vi "gas flow controller -- Pgg2.vi"(5 "gas flow, %":dbl=11.0, 6 "action":T3=enum."stop UP/DOWN", 7 "heater":dbl=11.0, 8 "gas flow controller ref":refnum<vi>, 10 "seconds":dbl=1.0) -> (0 "gas flow controller out":T1={"DOWN step (%)"=3.0, "below"=TRUE, "above"=FALSE, "check (min)"=11.0, "upper"=12.0, "lower"=3.0, "in range"=FALSE, "ramp step (%)"=0.1, "DOWN time (min)"=60.0, "UP time (min)"=60.0, "UP step (%)"=3.0, "set gas"=FALSE, "to"=90.0, "ramp UP"=FALSE, "ramp DOWN"=FALSE, "idle"=FALSE, "Control Gas"=TRUE, "state"=enum."ramp down", "ramp Up progress"={"(total # of ramp steps)"=30, "ramp time step (sec)"=120, "steps so far"=0, "state"=enum."ramp down"}, "ramp Down progress"={"(total # of ramp steps)"=30, "ramp time step (sec)"=120, "steps so far"=0, "state"=enum."ramp down"}, "last (min)"=90.0, "heater"=90.0, "gas, %"=90.0} {"last (min)" format="%3.3f"})   [LabVIEW 2014]
uses:
  gas flow controller action.ctl
  gas flow controller control.ctl
  gas flow control - progress.ctl
  gas flow controller state.ctl
  stack action -- control.ctl
  itc 503 box - control.ctl
  Q - not nan -- real.vi
  Q - not nan -- integer.vi
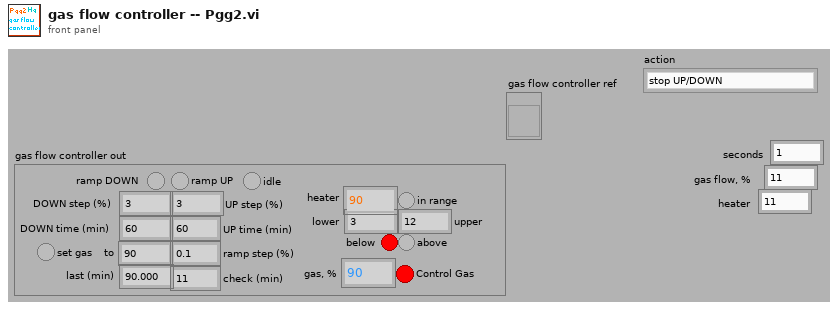
[diagram p1: front panel]
types:
  T1 = typedef "gas flow controller control.ctl" = cluster{"DOWN step (%)":dbl, "below":bool, "above":bool, "check (min)":dbl, "upper":dbl, "lower":dbl, "in range":bool, "ramp step (%)":dbl, "DOWN time (min)":dbl, "UP time (min)":dbl, "UP step (%)":dbl, "set gas":bool, "to":dbl, "ramp UP":bool, "ramp DOWN":bool, "idle":bool, "Control Gas":bool, "state":enum16{"normal", "ramp up", "ramp down"}, "ramp Up progress":T2, "ramp Down progress":T2, "last (min)":dbl, "heater":dbl, "gas, %":dbl}
  T2 = typedef "gas flow control - progress.ctl" = cluster{"(total # of ramp steps)":i32, "ramp time step (sec)":i32, "steps so far":i32, "state":enum16{"normal", "ramp up", "ramp down"}}
  T3 = typedef "gas flow controller action.ctl" = enum16{"check", "force UP", "stop UP/DOWN", "force DOWN", "init", "set gas to", "turn off", "turn on", "idle", "update parameters", "parse", "set gas"}
  T4 = typedef "gas flow controller state.ctl" = enum16{"normal", "ramp up", "ramp down"}
  T5 = typedef "stack action -- control.ctl" = enum16{"push", "pop", "check", "init"}
  T6 = typedef "itc 503 box - control.ctl" = enum16{"heater manual and zero", "heater auto", "upload D", "upload I", "upload P", "shut off", "init", "read sweep table", "disable", "enable", "read state", "set gas to", "stop sweep", "start sweep", "test", "set temperature to", "write sweep table", "-void", "set heater to"}
  T7 = typedef "comparison control.ctl" = enum16{"not a number", "above", "in range", "below"}
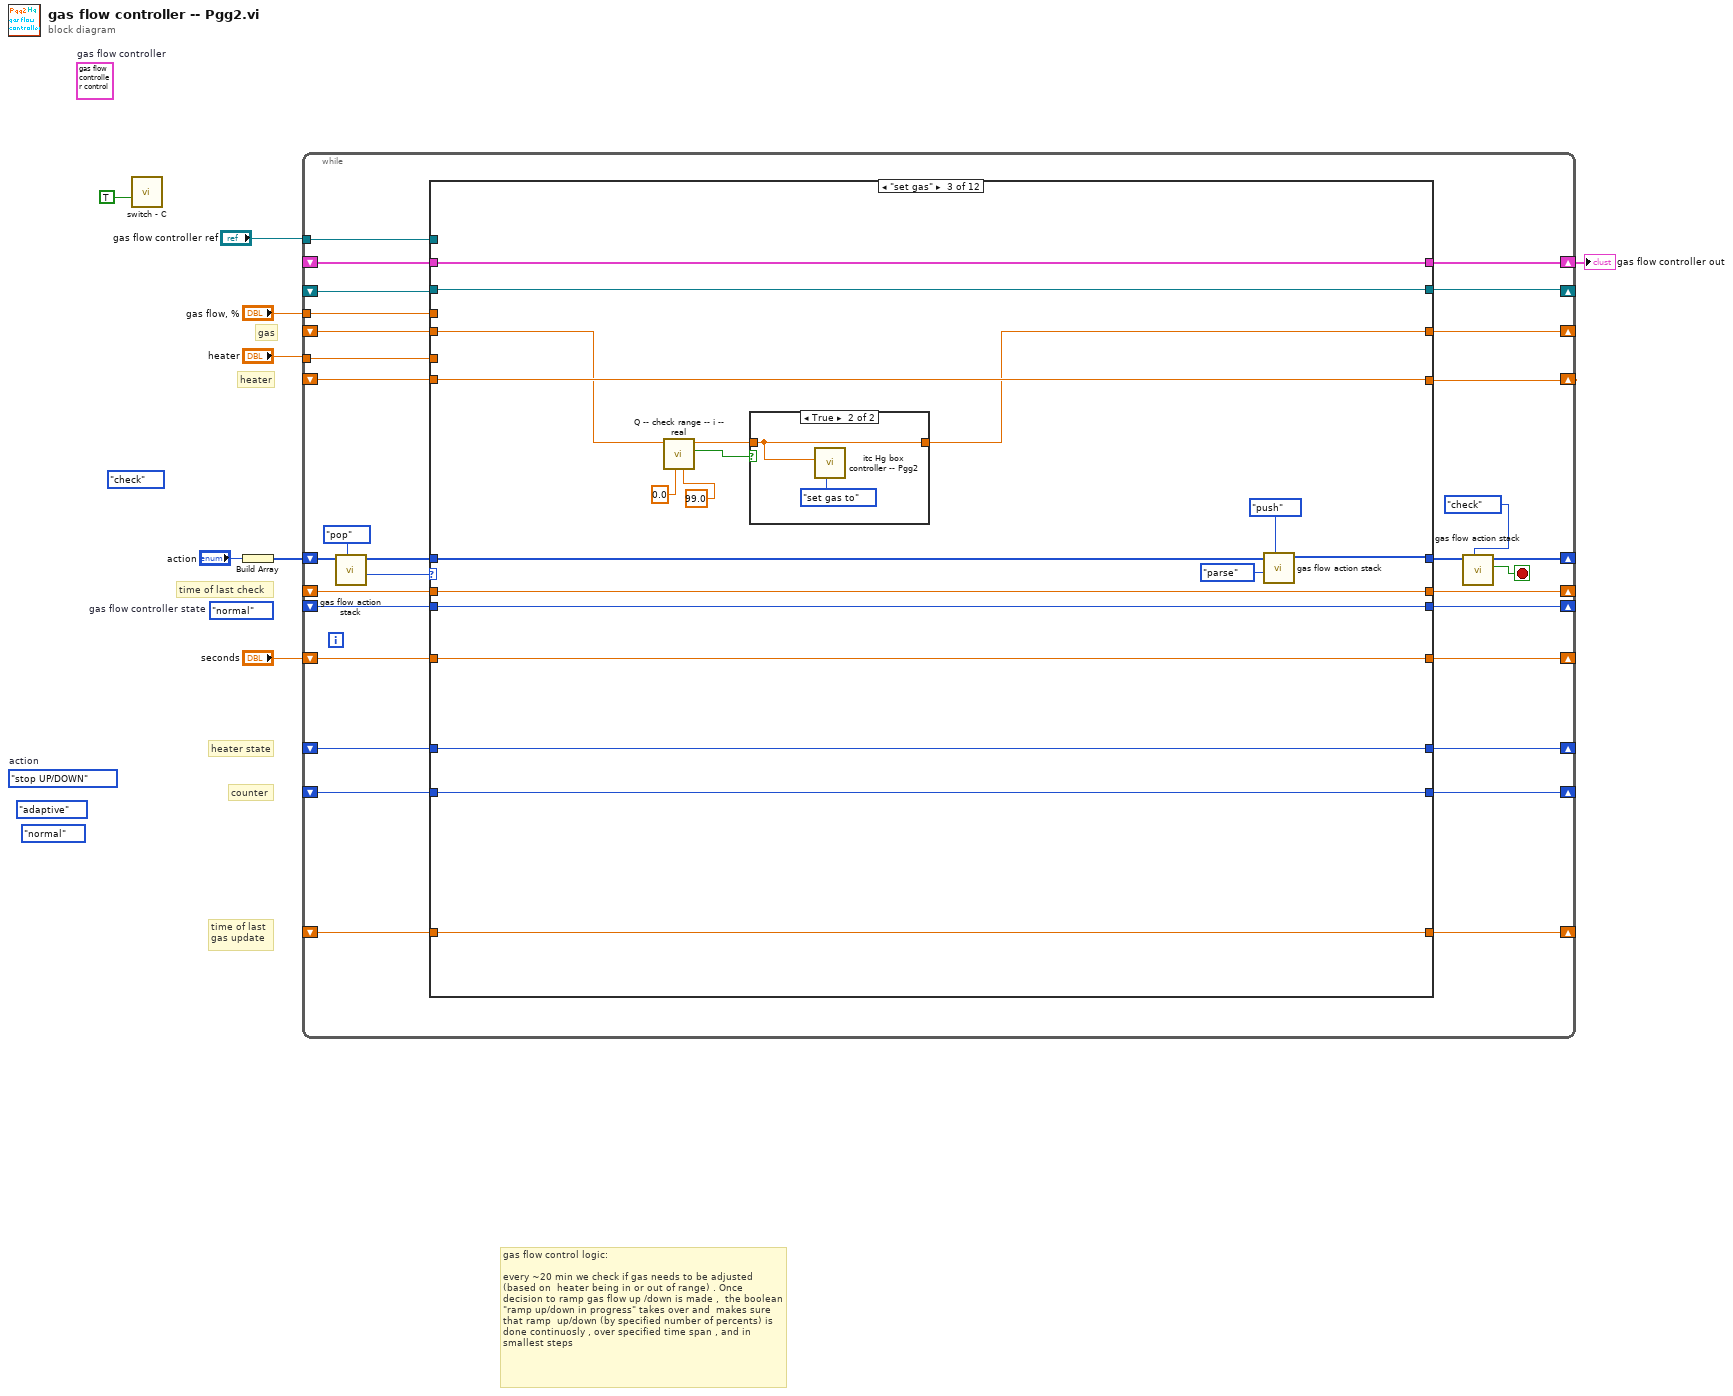
[diagram p0: block diagram]
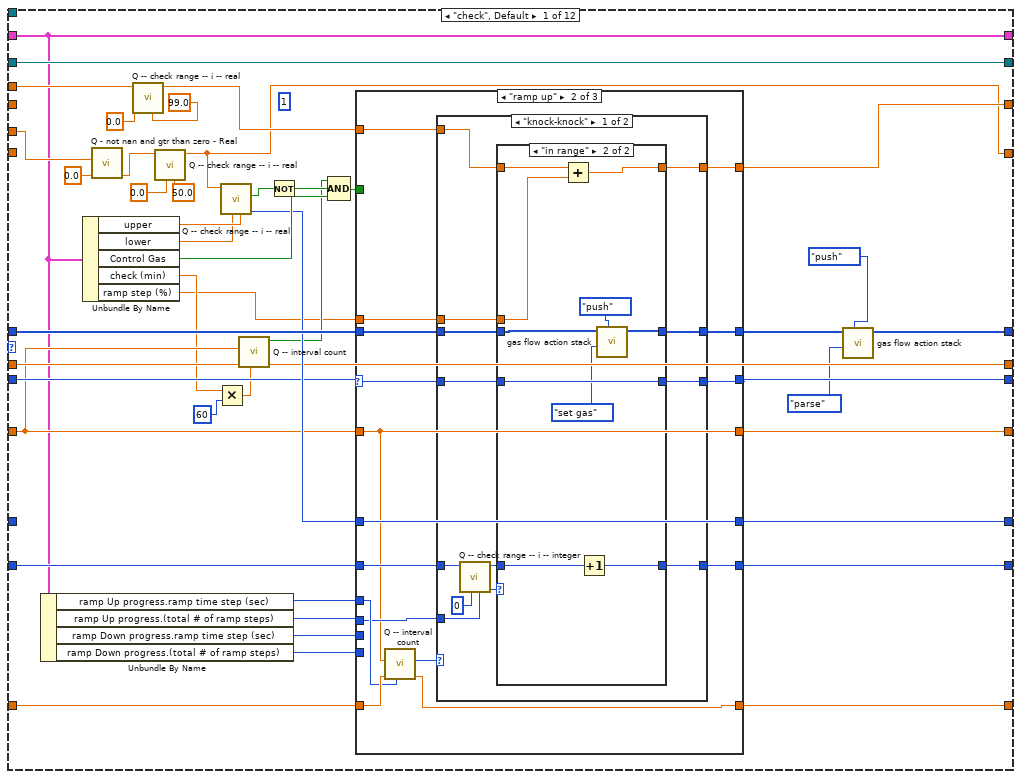
[diagram p2: hidden frame]
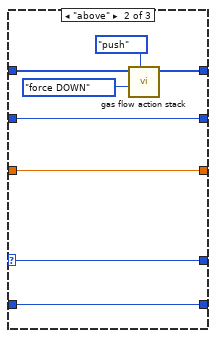
[diagram p5: hidden frame]
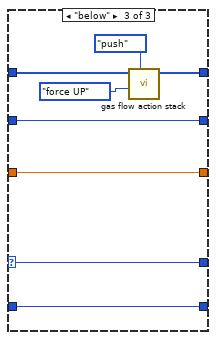
[diagram p6: hidden frame]
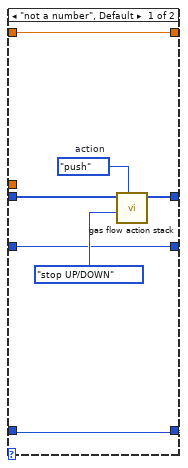
[diagram p7: hidden frame]
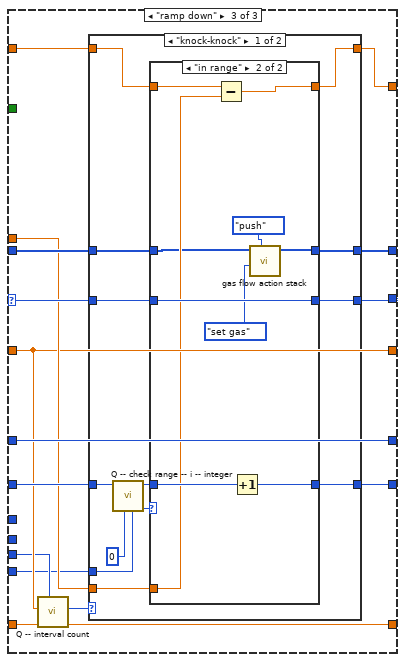
[diagram p9: hidden frame]
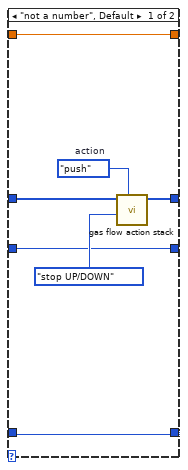
[diagram p10: hidden frame]
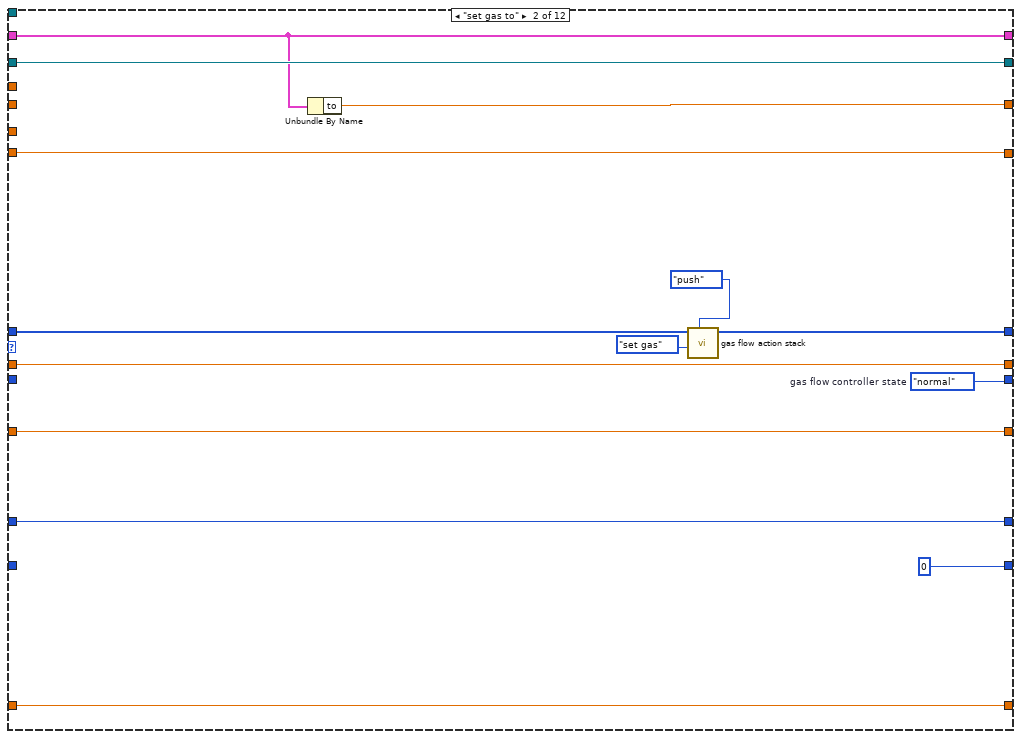
[diagram p12: hidden frame]
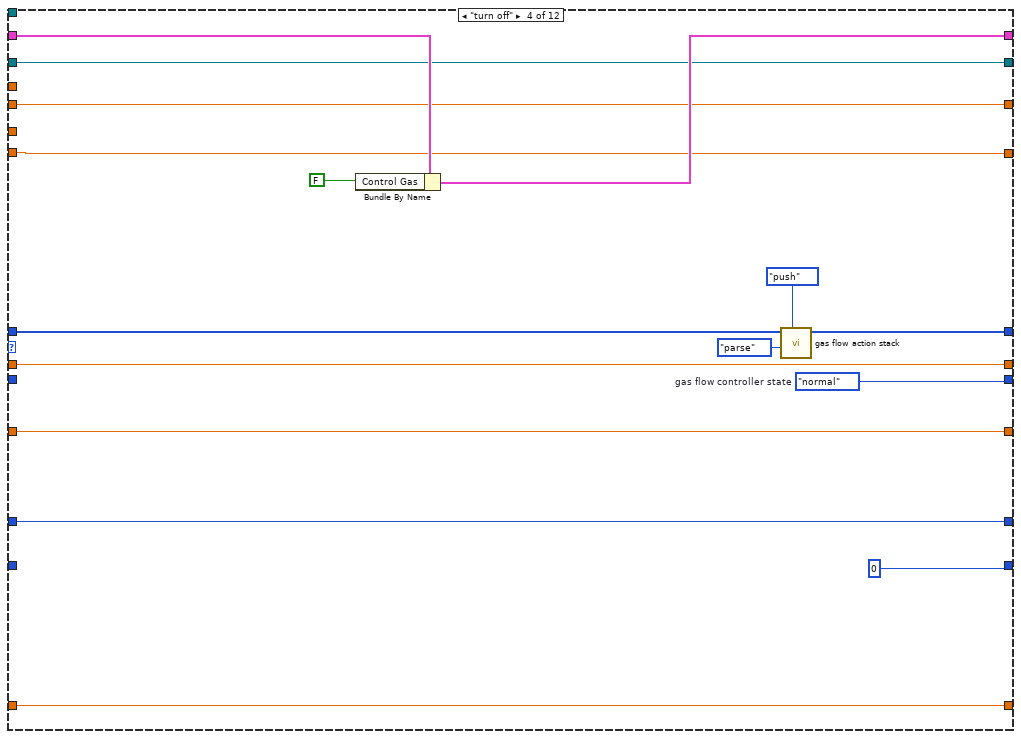
[diagram p14: hidden frame]
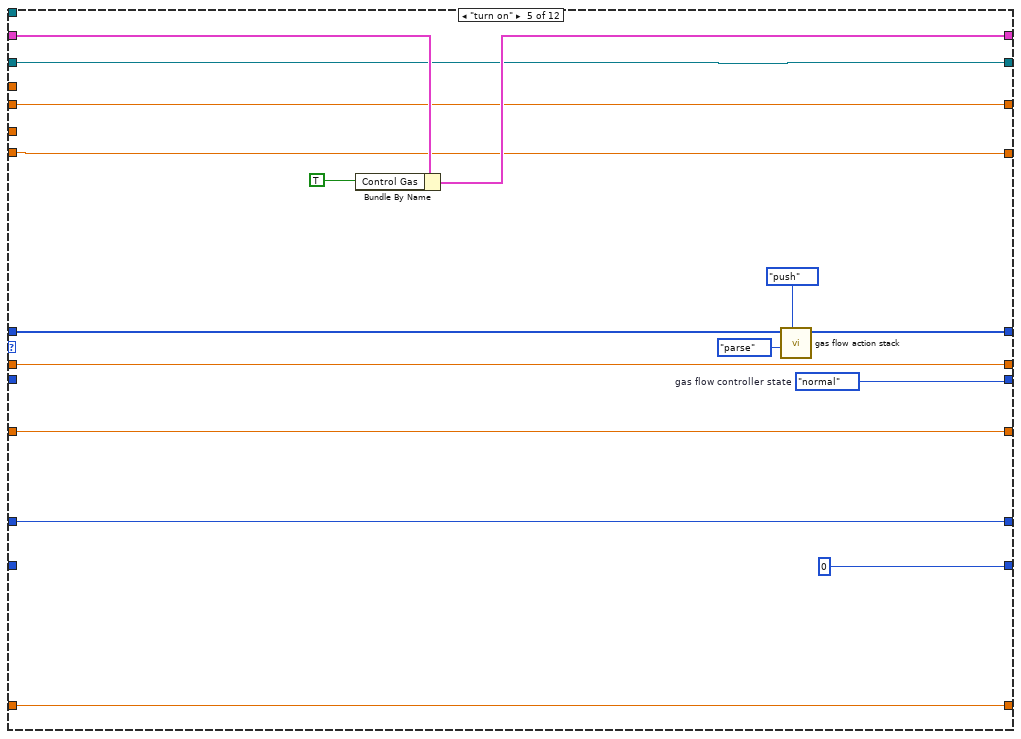
[diagram p15: hidden frame]
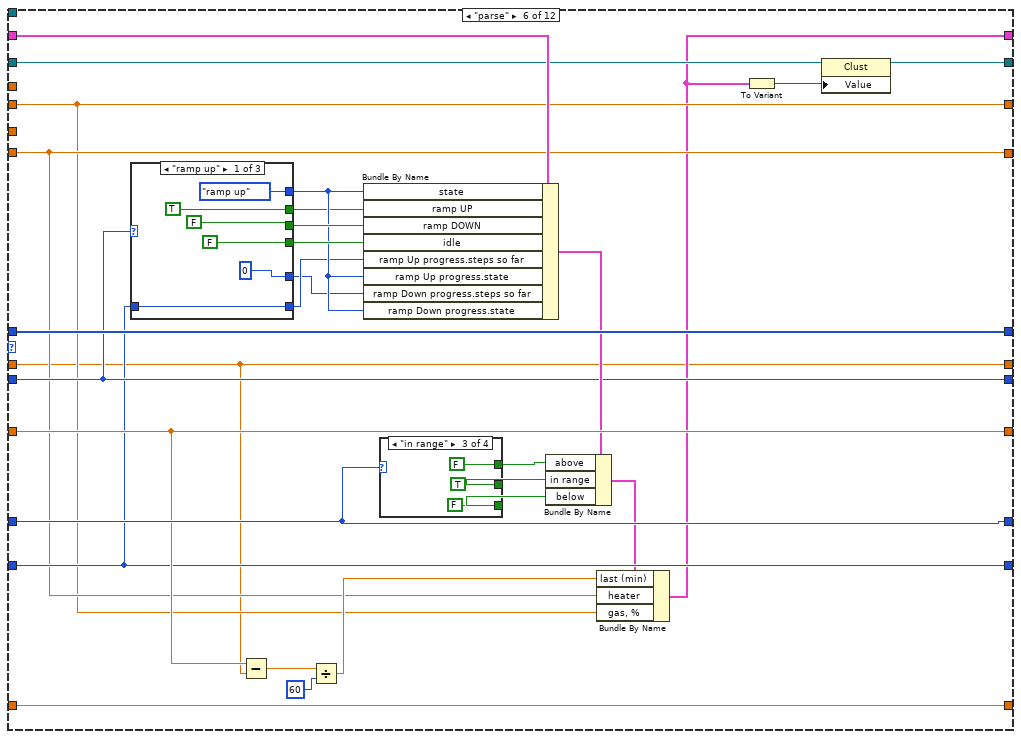
[diagram p16: hidden frame]
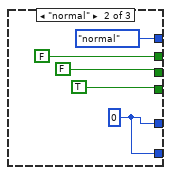
[diagram p17: hidden frame]
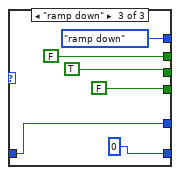
[diagram p18: hidden frame]
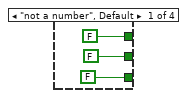
[diagram p19: hidden frame]
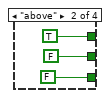
[diagram p20: hidden frame]
diagram:
  (unwired) gas_flow_controller_action."check" ("action")
  (unwired) T1 {"DOWN step (%)"=0.0, "below"=FALSE, "above"=FALSE, "check (min)"=0.0, "upper"=0.0, "lower"=0.0, "in range"=FALSE, "ramp step (%)"=0.0, "DOWN time (min)"=0.0, "UP time (min)"=0.0, "UP step (%)"=0.0, "set gas"=FALSE, "to"=0.0, "ramp UP"=FALSE, "ramp DOWN"=FALSE, "idle"=FALSE, "Control Gas"=FALSE, "state"=enum."normal", "ramp Up progress"={"(total # of ramp steps)"=0, "ramp time step (sec)"=0, "steps so far"=0, "state"=enum."normal"}, "ramp Down progress"={"(total # of ramp steps)"=0, "ramp time step (sec)"=0, "steps so far"=0, "state"=enum."normal"}, "last (min)"=0.0, "heater"=0.0, "gas, %"=0.0}  # gas flow controller
  (unwired) enum16{"normal", "ramp up", "ramp down"}."normal" ("state")
  (unwired) enum16{"first time", "uniform", "adaptive"}."adaptive" ("mode")
  (unwired) gas_flow_controller_state."normal"  # gas flow controller state
  (unwired) gas_flow_controller_action."stop UP/DOWN"  # action
  # "heater"
  # "time of last\ngas update"
  # "counter"
  # "heater state"
  # "gas"
  # "gas flow control logic: \n\nevery ~20 min we check if gas needs to be adjusted  (based on  heater being in or out of range) . Once  decision to ramp gas flow up /down is made ,  the boolean \"ramp up/down in progress\" takes over and  makes sure that ramp  up/down (by specified number of percents) is done continuosly , over specified time span , and in smallest steps"
  # "time of last check"
  n1 = call "switch - C.vi"("switch"=TRUE) -> ()  [unwired: 10 in, 1 out]
  n2 = Build Array("action") -> (w4:T3[])
  n3 = while {
    shift-right: [w39] -> w3
    shift-left: _ -> [w38]
    shift-right: [w20] -> _
    shift-left: _ -> [w17]
    tunnel: "gas flow, %" -> [w21]
    tunnel: "heater" -> [w37]
    shift-right: [w35] -> _
    shift-left: _ -> [w34]
    shift-right: [w33] -> _
    shift-left: _ -> [w32]
    shift-right: [w26] -> _
    shift-left: w4 -> [w31]
    shift-right: [w22] -> _
    shift-left: _ -> [w23]
    shift-right: [w19] -> _
    shift-left: _ -> [w18]
    shift-right: [w15] -> _
    shift-left: "seconds" -> [w36]
    shift-right: [w16] -> _
    shift-left: _ -> [w10]
    shift-right: [w14] -> _
    shift-left: _ -> [w13]
    shift-right: [w12] -> _
    shift-left: _ -> [w11]
    tunnel: "gas flow controller ref" -> [w9]
    stop <- w24 stop-if-true
    n4 = call "gas flow action stack.vi"("action"=stack_action_--_control."pop", "command stack"=w31) -> ("selector out"=w30:T3, "command stack out"=w28:T3[])  [unwired: 7 in, 1 out]
    n5 = case shown="\"set gas\"" w30 {
      tunnel: [w42 w236 w264 w281 w297 w304 w364 w411 w416 w437 w454 w469] -> w39
      tunnel: w38 -> [w42 w236 w264 w284 w300 w322 w369 w411 _ w437 w454 w469]
      tunnel: w37 -> [w47 _ _ _ _ _ _ _ _ _ _ _]
      tunnel: w36 -> [w64 w239 w262 w274 w290 w325 w375 w408 w421 w438 w443 w461]
      tunnel: [w53 w247 w266 w270 w286 w328 w380 w412 w420 w436 w455 w470] -> w35
      tunnel: w34 -> [w53 w247 w266 w270 w286 w306 w368 w412 _ w436 w455 w470]
      tunnel: [w73 w246 w265 w283 w299 w302 w378 w415 w431 w442 w445 w459] -> w33
      tunnel: w32 -> [w75 w246 w265 w283 w299 w302 w378 w415 w431 w442 _ _]
      tunnel: [w57 w243 w257 w279 w295 w329 w377 w403 w424 w435 w448 w463] -> w27
      tunnel: w28 -> [w78 w235 w256 w278 w294 w329 w377 w404 w425 w435 w449 w464]
      tunnel: w23 -> [w76 _ w254 _ _ w315 w376 _ _ w432 _ _]
      tunnel: [w70 w245 w254 w282 w298 w315 w376 w414 w430 w432 w457 w472] -> w22
      tunnel: w21 -> [w69 _ _ _ _ _ _ _ _ _ _ _]
      tunnel: [w49 w244 w248 w276 w292 w307 w370 w410 w428 w441 w453 w468] -> w20
      tunnel: [w48 w240 w263 w275 w291 w308 w371 w409 w427 w440 w452 w467] -> w19
      tunnel: w18 -> [_ w240 w263 w275 w291 w308 w371 w409 w427 w440 w452 w467]
      tunnel: w17 -> [_ _ w250 w276 w292 w307 w370 w410 w428 w441 w453 w468]
      tunnel: [w54 w238 w261 w273 w289 w327 w374 w407 w422 w439 w451 w466] -> w16
      tunnel: [w55 w239 w262 w274 w290 w325 w375 w408 w421 w438 w443 w461] -> w15
      tunnel: [w63 w237 w259 w272 w288 w326 w372 w405 w421 w434 w445 w459] -> w14
      tunnel: w13 -> [w62 w237 w259 w272 w288 w326 w372 w405 _ w434 w444 w458]
      tunnel: [w61 0 w260 0 0 w312 w373 0 0 w433 0 0] -> w12
      tunnel: w11 -> [w60 _ w260 _ _ w312 w373 _ _ w433 _ _]
      tunnel: w10 -> [_ w238 w261 w273 w289 w327 w374 w407 w422 w439 w451 w466]
      tunnel: w9 -> [_ _ _ _ _ _ _ _ w419 _ _ _]
      frame "check", Default {
        (unwired) 1
        n6 = Unbundle By Name(w42) -> ("ramp Up progress.ramp time step (sec)"=w52:i32, "ramp Up progress.(total # of ramp steps)"=w51:i32, "ramp Down progress.ramp time step (sec)"=w44:i32, "ramp Down progress.(total # of ramp steps)"=w43:i32)
        n7 = Unbundle By Name(w42) -> ("upper"=w82:dbl, "lower"=w81:dbl, "Control Gas"=w84:bool, "check (min)"=w41:dbl, "ramp step (%)"=w40:dbl)
        n8 = call "Q - not nan and gtr than zero - Real.vi"("default"=0.0 ("y"), "Numeric"=w47) -> ("out"=w45:dbl)  [unwired: 8 in, 1 out]
        n9 = call "Q -- check range -- i -- real.vi"("upper"=99.0 ("y"), "lower"=0.0 ("y"), "number"=w69) -> ("number in range"=w50:dbl)  [unwired: 6 in, 2 out]
        n10 = call "Q -- check range -- i -- real.vi"("upper"=50.0 ("y"), "lower"=0.0 ("y"), "number"=w45) -> ("number in range"=w48:dbl)  [unwired: 6 in, 2 out]
        n11 = Multiply(x=w41, y=60) -> (x*y=w74:dbl)
        n12 = call "Q -- check range -- i -- real.vi"("upper"=w82, "lower"=w81, "number"=w48) -> ("selector"=w77:T7, "in range?"=w80:bool)  [unwired: 6 in, 1 out]
        n13 = call "Q -- interval count.vi"("interval (sec)"=w74, "last time (sec)"=w75, "current time (sec)"=w64) -> ("last time out (sec)"=w73:dbl, "tic"=w71:bool)  [unwired: 5 in, 2 out]
        n14 = Not(x=w80) -> (.not. x?=w83:bool)
        n15 = Compound Arithmetic op=AND(w71, w83, w84) -> (w79:bool)
        n16 = case shown="\"ramp up\"" w76 {
          selector: w76 -> [w90 w142 w192]
          tunnel: w79 -> [w97 _ _]
          tunnel: w64 -> [w96 w134 w186]
          tunnel: [w85 w148 w198] -> w63
          tunnel: w62 -> [w85 w149 w199]
          tunnel: [w95 w145 w195] -> w58
          tunnel: w78 -> [w94 w144 w194]
          tunnel: w77 -> [w93 w140 w190]
          tunnel: [w92 w143 w193] -> w70
          tunnel: [w91 w146 w196] -> w61
          tunnel: w60 -> [w87 w147 w197]
          tunnel: [w89 w134 w186] -> w55
          tunnel: [w88 w140 w190] -> w54
          tunnel: w52 -> [_ w139 _]
          tunnel: w51 -> [_ w138 _]
          tunnel: w50 -> [w86 w137 w189]
          tunnel: w40 -> [_ w136 w188]
          tunnel: [w86 w135 w187] -> w49
          tunnel: w44 -> [_ _ w185]
          tunnel: w43 -> [_ _ w184]
          frame "normal", Default {
            n17 = case shown="False" w97 {
              tunnel: w96 -> [w100 w107]
              tunnel: [w102 w110] -> w95
              tunnel: w94 -> [w102 w111]
              tunnel: w93 -> [w99 w112]
              tunnel: [w101 w109] -> w92
              tunnel: w90 -> [w101 w108]
              tunnel: [w98 w106] -> w91
              tunnel: [w100 w105] -> w89
              tunnel: [w99 w104] -> w88
              tunnel: w87 -> [w98 w103]
              frame False {
              }
              frame True {
                n18 = case shown="\"not a number\", Default" w112 {
                  selector: w112 -> [w113 w119 w127]
                  tunnel: w111 -> [w117 w124 w132]
                  tunnel: [w117 w123 w131] -> w110
                  tunnel: [w116 w121 w129] -> w109
                  tunnel: w108 -> [w116 w121 w129]
                  tunnel: [w115 w120 w128] -> w105
                  tunnel: w107 -> [w115 w120 w128]
                  tunnel: [w114 w118 w126] -> w106
                  tunnel: [w113 w119 w127] -> w104
                  tunnel: w103 -> [w114 w118 w126]
                  frame "not a number", Default {
                  }
                  frame "above" {
                    n19 = call "gas flow action stack.vi"("action"=stack_action_--_control."push", "selector in"=gas_flow_controller_action."force DOWN" ("selector"), "command stack"=w124) -> ("command stack out"=w123:T3[])  [unwired: 6 in, 2 out]
                  }
                  frame "below" {
                    n20 = call "gas flow action stack.vi"("action"=stack_action_--_control."push", "selector in"=gas_flow_controller_action."force UP" ("selector"), "command stack"=w132) -> ("command stack out"=w131:T3[])  [unwired: 6 in, 2 out]
                  }
                }
              }
            }
          }
          frame "ramp up" {
            n21 = call "Q -- interval count.vi"("interval (sec)"=w139, "last time (sec)"=w149, "current time (sec)"=w134) -> ("last time out (sec)"=w148:dbl, "tic state"=w141:enum16{"knock-knock", "none"})  [unwired: 5 in, 2 out]
            n22 = case shown="\"knock-knock\"" w141 {
              tunnel: w147 -> [w154 w181]
              tunnel: [w158 w181] -> w146
              tunnel: [w162 w183] -> w145
              tunnel: w144 -> [w161 w183]
              tunnel: [w160 w182] -> w143
              tunnel: w142 -> [w159 w182]
              tunnel: w138 -> [w153 _]
              tunnel: w137 -> [w152 w180]
              tunnel: w136 -> [w151 _]
              tunnel: [w150 w180] -> w135
              frame "knock-knock" {
                n23 = call "Q -- check range -- i -- integer.vi"("upper"=w153, "lower"=0, "number"=w154) -> ("selector"=w156:T7, "number in range"=w155:i32)  [unwired: 6 in, 1 out]
                n24 = case shown="\"in range\"" w156 {
                  tunnel: [w167 w171] -> w162
                  tunnel: w161 -> [w168 w172]
                  tunnel: [w165 w179] -> w160
                  tunnel: w159 -> [w165 w179]
                  tunnel: w155 -> [w164 w178]
                  tunnel: [w164 w177] -> w158
                  tunnel: w152 -> [w163 w176]
                  tunnel: w151 -> [_ w175]
                  tunnel: [w163 w174] -> w150
                  frame "not a number", Default {
                    w169 = stack_action_--_control."push"  # action
                    n25 = call "gas flow action stack.vi"("action"=w169, "selector in"=gas_flow_controller_action."stop UP/DOWN" ("selector"), "command stack"=w168) -> ("command stack out"=w167:T3[])  [unwired: 6 in, 2 out]
                  }
                  frame "in range" {
                    n26 = Add(x=w176, y=w175) -> (x+y=w174:dbl)
                    n27 = Increment(x=w178) -> (x+1=w177:i32)
                    n28 = call "gas flow action stack.vi"("action"=stack_action_--_control."push", "selector in"=gas_flow_controller_action."set gas" ("selector"), "command stack"=w172) -> ("command stack out"=w171:T3[])  [unwired: 6 in, 2 out]
                  }
                }
              }
              frame "none", Default {
              }
            }
          }
          frame "ramp down" {
            n29 = call "Q -- interval count.vi"("interval (sec)"=w185, "last time (sec)"=w199, "current time (sec)"=w186) -> ("last time out (sec)"=w198:dbl, "tic state"=w191:enum16{"knock-knock", "none"})  [unwired: 5 in, 2 out]
            n30 = case shown="\"knock-knock\"" w191 {
              tunnel: w197 -> [w204 w231]
              tunnel: [w208 w231] -> w196
              tunnel: [w212 w233] -> w195
              tunnel: w194 -> [w211 w233]
              tunnel: [w210 w232] -> w193
              tunnel: w192 -> [w209 w232]
              tunnel: w184 -> [w203 _]
              tunnel: w189 -> [w202 w230]
              tunnel: w188 -> [w201 _]
              tunnel: [w200 w230] -> w187
              frame "knock-knock" {
                n31 = call "Q -- check range -- i -- integer.vi"("upper"=w203, "lower"=0, "number"=w204) -> ("selector"=w206:T7, "number in range"=w205:i32)  [unwired: 6 in, 1 out]
                n32 = case shown="\"in range\"" w206 {
                  tunnel: [w217 w221] -> w212
                  tunnel: w211 -> [w218 w222]
                  tunnel: [w215 w229] -> w210
                  tunnel: w209 -> [w215 w229]
                  tunnel: w205 -> [w214 w228]
                  tunnel: [w214 w227] -> w208
                  tunnel: w202 -> [w213 w226]
                  tunnel: w201 -> [_ w225]
                  tunnel: [w213 w224] -> w200
                  frame "not a number", Default {
                    w219 = stack_action_--_control."push"  # action
                    n33 = call "gas flow action stack.vi"("action"=w219, "selector in"=gas_flow_controller_action."stop UP/DOWN" ("selector"), "command stack"=w218) -> ("command stack out"=w217:T3[])  [unwired: 6 in, 2 out]
                  }
                  frame "in range" {
                    n34 = Subtract(x=w226, y=w225) -> (x-y=w224:dbl)
                    n35 = Increment(x=w228) -> (x+1=w227:i32)
                    n36 = call "gas flow action stack.vi"("action"=stack_action_--_control."push", "selector in"=gas_flow_controller_action."set gas" ("selector"), "command stack"=w222) -> ("command stack out"=w221:T3[])  [unwired: 6 in, 2 out]
                  }
                }
              }
              frame "none", Default {
              }
            }
          }
        }
        n37 = call "gas flow action stack.vi"("action"=stack_action_--_control."push", "selector in"=gas_flow_controller_action."parse" ("selector"), "command stack"=w58) -> ("command stack out"=w57:T3[])  [unwired: 6 in, 2 out]
      }
      frame "set gas to" {
        w245 = gas_flow_controller_state."normal"  # gas flow controller state
        n38 = Unbundle By Name(w236) -> ("to"=w244:dbl)
        n39 = call "gas flow action stack.vi"("action"=stack_action_--_control."push", "selector in"=gas_flow_controller_action."set gas" ("selector"), "command stack"=w235) -> ("command stack out"=w243:T3[])  [unwired: 6 in, 2 out]
      }
      frame "set gas" {
        n40 = call "Q -- check range -- i -- real.vi"("upper"=99.0 ("y"), "lower"=0.0 ("y"), "number"=w250) -> ("in range?"=w251:bool, "number in range"=w249:dbl)  [unwired: 6 in, 1 out]
        n41 = case shown="True" w251 {
          tunnel: [w267 w268] -> w248
          tunnel: w249 -> [w267 w268]
          frame False {
          }
          frame True {
            n42 = call "itc Hg box controller -- Pgg2.vi"("itc box action"=itc_503_box_-_control."set gas to", "input"=w268) -> ()  [unwired: 7 in, 3 out]
          }
        }
        n43 = call "gas flow action stack.vi"("action"=stack_action_--_control."push", "selector in"=gas_flow_controller_action."parse" ("selector"), "command stack"=w256) -> ("command stack out"=w257:T3[])  [unwired: 6 in, 2 out]
      }
      frame "turn off" {
        w282 = gas_flow_controller_state."normal"  # gas flow controller state
        n44 = Bundle By Name(cluster=w284, "Control Gas"=FALSE) -> (w281:T1)
        n45 = call "gas flow action stack.vi"("action"=stack_action_--_control."push", "selector in"=gas_flow_controller_action."parse" ("selector"), "command stack"=w278) -> ("command stack out"=w279:T3[])  [unwired: 6 in, 2 out]
      }
      frame "turn on" {
        w298 = gas_flow_controller_state."normal"  # gas flow controller state
        n46 = Bundle By Name(cluster=w300, "Control Gas"=TRUE) -> (w297:T1)
        n47 = call "gas flow action stack.vi"("action"=stack_action_--_control."push", "selector in"=gas_flow_controller_action."parse" ("selector"), "command stack"=w294) -> ("command stack out"=w295:T3[])  [unwired: 6 in, 2 out]
      }
      frame "parse" {
        n48 = case shown="\"ramp up\"" w315 {
          tunnel: [TRUE FALSE FALSE] -> w303
          tunnel: [FALSE FALSE TRUE] -> w321
          tunnel: [FALSE TRUE FALSE] -> w320
          tunnel: [enum16{"normal", "ramp up", "ramp down"}."ramp up" ("state") enum16{"normal", "ramp up", "ramp down"}."normal" ("state") enum16{"normal", "ramp up", "ramp down"}."ramp down" ("state")] -> w314
          tunnel: [0 w336 w341] -> w311
          tunnel: [w330 w336 0] -> w313
          tunnel: w312 -> [w330 _ w341]
          frame "ramp up" {
          }
          frame "normal" {
            w336 = 0
          }
          frame "ramp down" {
          }
        }
        n49 = Subtract(x=w325, y=w302) -> (x-y=w323:dbl)
        n50 = Divide(x=w323, y=60) -> (x/y=w309:dbl)
        n51 = Bundle By Name(cluster=w322, "state"=w314, "ramp UP"=w303, "ramp DOWN"=w321, "idle"=w320, "ramp Up progress.steps so far"=w313, "ramp Up progress.state"=w314, "ramp Down progress.steps so far"=w311, "ramp Down progress.state"=w314) -> (w316:T1)
        n52 = case shown="\"in range\"" w327 {
          tunnel: [FALSE TRUE FALSE FALSE] -> w319
          tunnel: [FALSE FALSE TRUE FALSE] -> w318
          tunnel: [FALSE FALSE FALSE TRUE] -> w317
          frame "not a number", Default {
          }
          frame "above" {
          }
          frame "in range" {
          }
          frame "below" {
          }
        }
        n53 = Bundle By Name(cluster=w316, "above"=w319, "in range"=w318, "below"=w317) -> (w310:T1)
        n54 = Bundle By Name(cluster=w310, "last (min)"=w309, "heater"=w308, "gas, %"=w307) -> (w304:T1)
        n55 = To Variant(anything=w304) -> (Variant=w305:variant)
        n56 = property class="Clust"(reference=w306, "Value"=w305) -> (reference out=w328:refnum<vi>)  [unwired: 1 in, 1 out]
      }
      frame "update parameters" {
        w365 = T1 {"DOWN step (%)"=0.0, "below"=FALSE, "above"=FALSE, "check (min)"=0.0, "upper"=0.0, "lower"=0.0, "in range"=FALSE, "ramp step (%)"=0.0, "DOWN time (min)"=0.0, "UP time (min)"=0.0, "UP step (%)"=0.0, "set gas"=FALSE, "to"=0.0, "ramp UP"=FALSE, "ramp DOWN"=FALSE, "idle"=FALSE, "Control Gas"=FALSE, "state"=enum."normal", "ramp Up progress"={"(total # of ramp steps)"=0, "ramp time step (sec)"=0, "steps so far"=0, "state"=enum."normal"}, "ramp Down progress"={"(total # of ramp steps)"=0, "ramp time step (sec)"=0, "steps so far"=0, "state"=enum."normal"}, "last (min)"=0.0, "heater"=0.0, "gas, %"=0.0}  # gas flow controller
        # "update  parameters"
        n57 = property class="Clust"(reference=w368) -> (reference out=w367:refnum<vi>, "Value"=w366:variant)  [unwired: 1 in, 1 out]
        n58 = Variant To Data(type=w365, Variant=w366) -> (data=w361:T1)  [unwired: 1 in, 1 out]
        n59 = Unbundle By Name(w361) -> ("DOWN step (%)"=w387:dbl, "DOWN time (min)"=w386:dbl)
        n60 = Unbundle By Name(w361) -> ("ramp step (%)"=w360:dbl)
        n61 = Unbundle By Name(w361) -> ("UP step (%)"=w379:dbl, "UP time (min)"=w388:dbl)
        n62 = Divide(x=w379, y=w360) -> (x/y=w401:dbl)
        n63 = Divide(x=w387, y=w360) -> (x/y=w394:dbl)
        n64 = Multiply(x=w388, y=60) -> (x*y=w399:dbl)
        n65 = Multiply(x=w386, y=60) -> (x*y=w392:dbl)
        n66 = Round Toward +Infinity(x=w399) -> (ceil(x): smallest int >= x=w398:dbl)
        n67 = Round Toward +Infinity(x=w401) -> (ceil(x): smallest int >= x=w400:dbl)
        n68 = Round Toward +Infinity(x=w394) -> (ceil(x): smallest int >= x=w393:dbl)
        n69 = Round Toward +Infinity(x=w392) -> (ceil(x): smallest int >= x=w391:dbl)
        n70 = To Long Integer(number=w398) -> (32bit integer=w396:i32)
        n71 = To Long Integer(number=w400) -> (32bit integer=w395:i32)
        n72 = To Long Integer(number=w393) -> (32bit integer=w384:i32)
        n73 = To Long Integer(number=w391) -> (32bit integer=w389:i32)
        n74 = Unbundle By Name(w361) -> ("to"=w383:dbl, "upper"=w382:dbl, "lower"=w381:dbl, "check (min)"=w359:dbl)
        n75 = Quotient & Remainder(x=w396, y=w395) -> (floor(x/y)=w362:i32)  [unwired: 1 out]
        n76 = Quotient & Remainder(x=w389, y=w384) -> (floor(x/y)=w385:i32)  [unwired: 1 out]
        n77 = Bundle By Name(cluster=w369, "ramp Up progress.(total # of ramp steps)"=w395, "ramp Up progress.ramp time step (sec)"=w362, "UP step (%)"=w379, "UP time (min)"=w388, "ramp step (%)"=w360, "DOWN step (%)"=w387, "DOWN time (min)"=w386, "ramp Down progress.(total # of ramp steps)"=w384, "ramp Down progress.ramp time step (sec)"=w385, "to"=w383, "upper"=w382, "lower"=w381, "check (min)"=w359) -> (w364:T1)
        n78 = To Variant(anything=w364) -> (Variant=w363:variant)
        n79 = property class="Clust"(reference=w367, "Value"=w363) -> (reference out=w380:refnum<vi>)  [unwired: 1 in, 1 out]
      }
      frame "stop UP/DOWN" {
        w414 = gas_flow_controller_state."normal"  # gas flow controller state
        n80 = call "gas flow action stack.vi"("action"=stack_action_--_control."push", "selector in"=gas_flow_controller_action."parse" ("selector"), "command stack"=w404) -> ("command stack out"=w403:T3[])  [unwired: 6 in, 2 out]
      }
      frame "init" {
        w417 = T1 {"DOWN step (%)"=0.0, "below"=FALSE, "above"=FALSE, "check (min)"=0.0, "upper"=0.0, "lower"=0.0, "in range"=FALSE, "ramp step (%)"=0.0, "DOWN time (min)"=0.0, "UP time (min)"=0.0, "UP step (%)"=0.0, "set gas"=FALSE, "to"=0.0, "ramp UP"=FALSE, "ramp DOWN"=FALSE, "idle"=FALSE, "Control Gas"=FALSE, "state"=enum."normal", "ramp Up progress"={"(total # of ramp steps)"=0, "ramp time step (sec)"=0, "steps so far"=0, "state"=enum."normal"}, "ramp Down progress"={"(total # of ramp steps)"=0, "ramp time step (sec)"=0, "steps so far"=0, "state"=enum."normal"}, "last (min)"=0.0, "heater"=0.0, "gas, %"=0.0}  # gas flow controller
        w430 = gas_flow_controller_state."normal"  # gas flow controller state
        n81 = property class="Clust"(reference=w419) -> (reference out=w420:refnum<vi>, "Value"=w418:variant)  [unwired: 1 in, 1 out]
        n82 = Variant To Data(type=w417, Variant=w418) -> (data=w416:T1)  [unwired: 1 in, 1 out]
        n83 = call "gas flow action stack.vi"("action"=stack_action_--_control."push", "selector in"=gas_flow_controller_action."parse" ("selector"), "command stack"=w425) -> ("command stack out"=w424:T3[])  [unwired: 6 in, 2 out]
      }
      frame "idle" {
      }
      frame "force DOWN" {
        w457 = gas_flow_controller_state."ramp down"  # gas flow controller state
        n84 = Subtract(x=w444, y=10000) -> (x-y=w445:dbl)
        n85 = call "gas flow action stack.vi"("action"=stack_action_--_control."push", "selector in"=gas_flow_controller_action."parse" ("selector"), "command stack"=w449) -> ("command stack out"=w448:T3[])  [unwired: 6 in, 2 out]
      }
      frame "force UP" {
        w472 = gas_flow_controller_state."ramp up"  # gas flow controller state
        n86 = Subtract(x=w458, y=10000) -> (x-y=w459:dbl)
        n87 = call "gas flow action stack.vi"("action"=stack_action_--_control."push", "selector in"=gas_flow_controller_action."parse" ("selector"), "command stack"=w464) -> ("command stack out"=w463:T3[])  [unwired: 6 in, 2 out]
      }
    }
    n88 = call "gas flow action stack.vi"("action"=stack_action_--_control."check", "command stack"=w27) -> ("stack is empty ?"=w24:bool, "command stack out"=w26:T3[])  [unwired: 7 in, 1 out]
  }
  "gas flow controller out" <- w3
